vi "Calculate Built Version.vi"(0 "NI Build Specification_LV in":refnum<class "NI Build Specification_LV.lvclass">, 11 "error in (no error)":errorcluster) -> (4 "NI Build Specification_LV out":refnum<class "NI Build Specification_LV.lvclass">, 15 "error out":errorcluster)   [LabVIEW 2017, in "CL_G3_VIComponentBuilder.lvlib" / "NI Build Specification_LV.lvclass"]
uses:
  NI Build Specification_LV.lvclass
  C:/builds/Component BuilderBT/SrcDist/Exports/Exports/Export.lvclass
  NI Build Specification_LV.lvclass/NI Build Specification_LV.ctl
  Exports/Export.lvclass/Export.ctl
  Accessors/Read Project Reference.vi
  Accessors/Read Export's Build Spec Name.vi
  Accessors/Read Target Name Containing Build Specs to Build.vi
  Exports/Accessors/Write Built Version.vi
  <vilib>/AppBuilder/AB_API_Simple/Get Build Specification Version (project reference).vi
  <vilib>/AppBuilder/AB_API_Simple/NI_App_Builder_API.lvlib
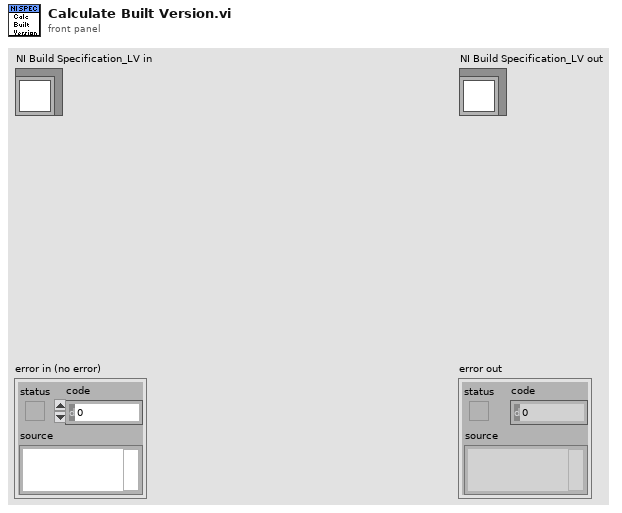
[diagram p1: front panel]
types:
  T1 = typedef "NI_App_Builder_API.lvlib/Build Specification Version.ctl" = cluster{"Major":u16, "Minor":u16, "Fix":u16, "Build":u16}
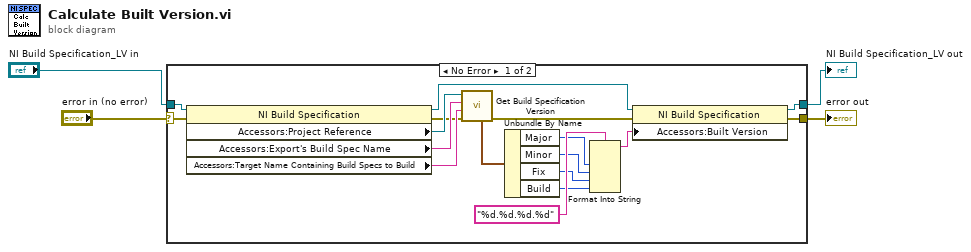
[diagram p0: block diagram]
diagram:
  n1 = case shown="No Error" "error in (no error)" {
    selector: "error in (no error)" -> [w18 w22]
    tunnel: "NI Build Specification_LV in" -> [w21 w23]
    tunnel: [w20 w23] -> w3
    tunnel: [w19 w22] -> w1
    frame No Error {
      n2 = property class="NI Build Specification"(reference=w21, error in=w18) -> (reference out=w13:refnum<class "NI Build Specification_LV.lvclass">, error out=w12:errorcluster, "Accessors:Project Reference"=w17:refnum<vi>, "Accessors:Export's Build Spec Name"=w15:string, "Accessors:Target Name Containing Build Specs to Build"=w16:string)
      n3 = call-poly <vilib>:"Get Build Specification Version.vi"("error in (no error)"=w12, "Name of target (My Computer)"=w16, "Name of build specification"=w15, "Project reference"=w17) -> ("error out"=w14:errorcluster, "Build Specification Version"=w5:T1)  [unwired: 5 in, 1 out]
      n4 = Unbundle By Name(w5) -> ("Major"=w10:u16, "Minor"=w9:u16, "Fix"=w8:u16, "Build"=w7:u16)
      n5 = Format Into String(format string="%d.%d.%d.%d", w10, w9, w8, w7) -> (resulting string=w6:string)  [unwired: 2 in, 1 out]
      n6 = property class="NI Build Specification"(reference=w13, error in=w14, "Accessors:Built Version"=w6) -> (reference out=w20:refnum<class "NI Build Specification_LV.lvclass">, error out=w19:errorcluster)
    }
    frame Error {
    }
  }
  "error out" <- w1
  "NI Build Specification_LV out" <- w3
